vi "34401 - Config Measurement.vi"(0 "address":string, 1 "Manual Res. (1:5.5 Digits)":u16(ring)=1 items=["4.5 Digits", "5.5 Digits", "6.5 Digits"], 2 "Function (0:V DC)":u16(ring) items=["DC Voltage", "AC Voltage", "2--Wire Resistance", "4-Wire Resistance", "DC Current", "AC Current", "Frequency", "Period", "Continuity", "Diode Checking", "VDC: VDC Ratio"], 3 "AC Filter (1:Medium)":u16(ring)=1 items=["Slow", "Medium", "Fast"], 5 "Fixed DC Input Res. (T:On)":bool=TRUE, 7 "Manual Int. (0:Default)":u16(ring) items=["Default", "0.02 PLCs", "0.2 PLC", "1 PLCs", "10 PLCs", "100 PLCs"], 9 "Manual Apr. (0:Default)":u16(ring) items=["Default", "0.01 Sec", "0.1 Sec", "1 Sec"], 11 "error in (no error)":errorcluster, 12 "Ran/Res/Int/Apr (T:Auto)":bool=TRUE, 13 "Autozero (F:Off)":bool, 14 "Manual Range (0.00)":dbl min=0.0 format="%.2f") -> (15 "error out":errorcluster)   [LabVIEW 2014]
doc: "Configures the range, resolution, and other settings for the multimeter measurement."
panel:
  # "Auto"
  # "Manual"
  # "ON\nOFF"
  # "ON\nOFF"
  # "Note - Manually setting either the integration or aperture overrides the manual resolution settings."
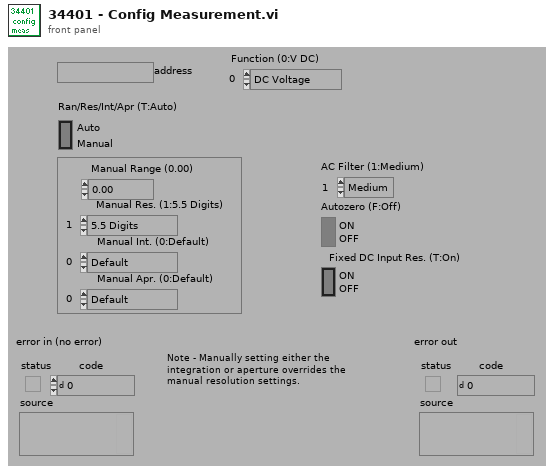
[diagram p1: front panel]
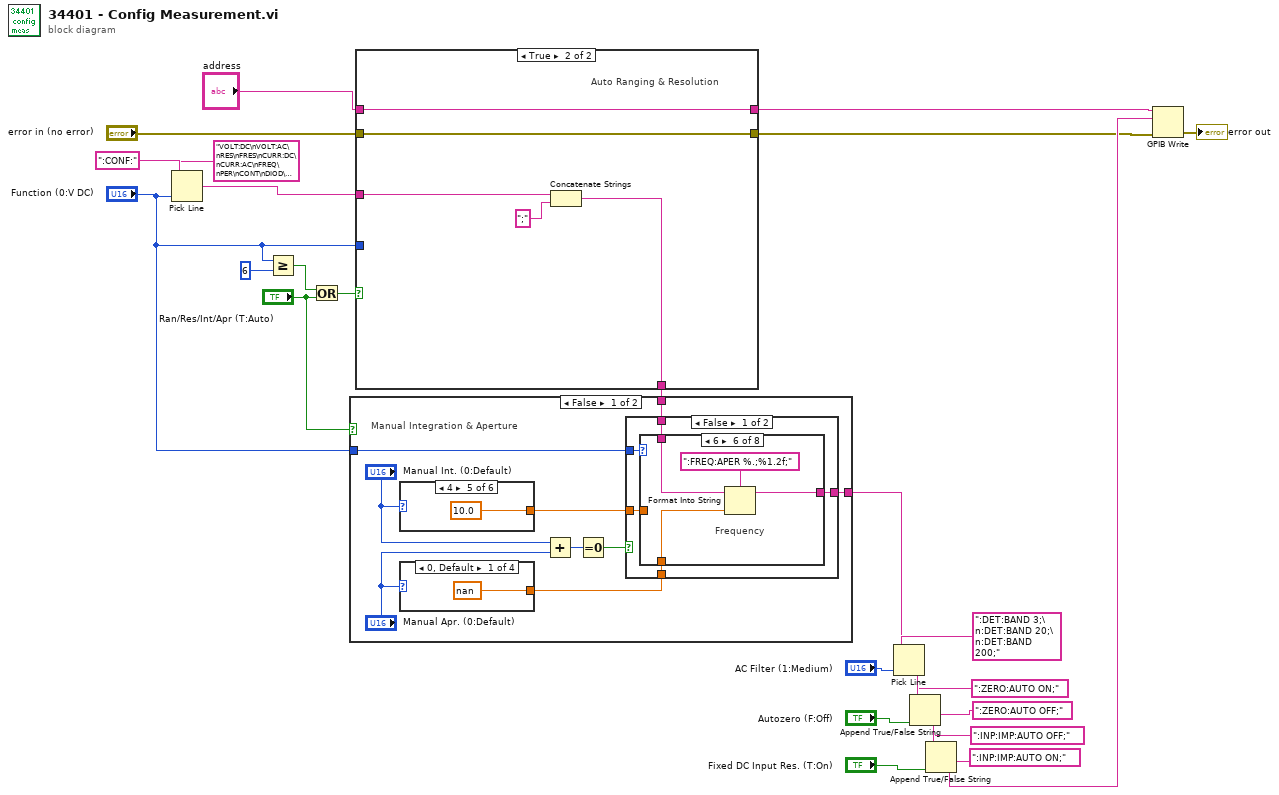
[diagram p0: block diagram]
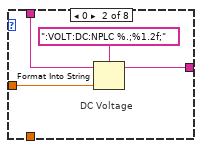
[diagram p3: hidden frame]
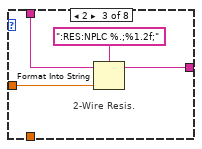
[diagram p4: hidden frame]
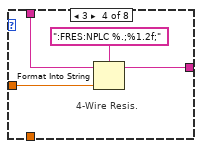
[diagram p5: hidden frame]
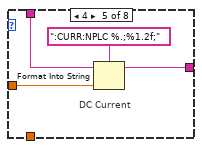
[diagram p6: hidden frame]
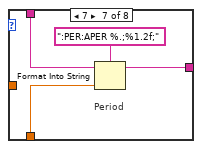
[diagram p7: hidden frame]
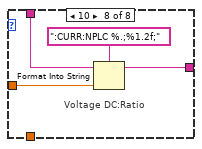
[diagram p8: hidden frame]
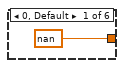
[diagram p10: hidden frame]
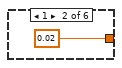
[diagram p11: hidden frame]
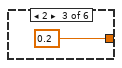
[diagram p12: hidden frame]
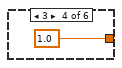
[diagram p13: hidden frame]
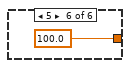
[diagram p14: hidden frame]
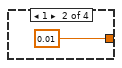
[diagram p15: hidden frame]
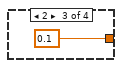
[diagram p16: hidden frame]
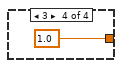
[diagram p17: hidden frame]
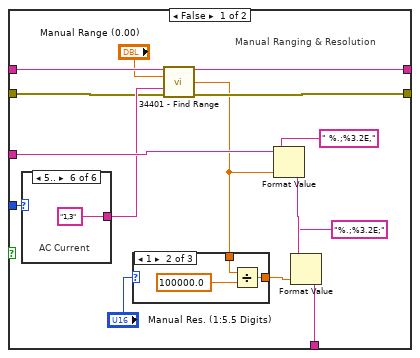
[diagram p19: hidden frame]
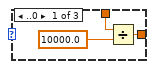
[diagram p20: hidden frame]
diagram:
  n1 = Pick Line(string ("")=":CONF:", multi-line string="VOLT:DC\nVOLT:AC\nRES\nFRES\nCURR:DC\nCURR:AC\nFREQ\nPER\nCONT\nDIOD\nVOLT:DC:RAT", line index="Function (0:V DC)") -> (output string=w21:string)
  n2 = Greater Or Equal?(x="Function (0:V DC)", y=u16 6) -> (x >= y?=w23:bool)
  n3 = Or(x=w23, y="Ran/Res/Int/Apr (T:Auto)") -> (x .or. y?=w22:bool)
  n4 = case shown="True" w22 {
    tunnel: w21 -> [w40 w61]
    tunnel: "Function (0:V DC)" -> [w41 _]
    tunnel: [w34 w59] -> w9
    tunnel: "error in (no error)" -> [w30 w58]
    tunnel: [w27 w57] -> w3
    tunnel: [w29 w58] -> w1
    tunnel: "address" -> [w33 w57]
    frame False {
      # "Manual Ranging & Resolution"
      n5 = case shown="5.." w41 {
        tunnel: [".1,1,10,100,1000" ".1,1,10,100,1000" "1E2,1E3,1E4,1E5,1E6,1E7,1E8" "1E2,1E3,1E4,1E5,1E6,1E7,1E8" ".01,.1,1,3" "1,3"] -> w31
        frame ..0 {
          # "DC Voltage"
        }
        frame 1 {
          # "AC Voltage"
        }
        frame 2 {
          # "2-Wire Resis."
        }
        frame 3 {
          # "4-Wire Resis."
        }
        frame 4 {
          # "DC Current"
        }
        frame 5.. {
          # "AC Current"
        }
      }
      n6 = call "34401 - Find Range.vi"("address"=w33, "Number to Range (0.00)"="Manual Range (0.00)", "Numeric Data (Empty)"=w31, "error in (no error)"=w30) -> ("dup address"=w27:string, "Ranged Number"=w28:dbl, "error out"=w29:errorcluster)  [unwired: 7 in, 2 out]
      n7 = case shown="1" "Manual Res. (1:5.5 Digits)" {
        tunnel: w28 -> [w43 w46 w49]
        tunnel: [w42 w45 w48] -> w38
        frame ..0 {
          n8 = Divide(x=w43, y=10000.0) -> (x/y=w42:dbl)
        }
        frame 1 {
          n9 = Divide(x=w46, y=100000.0) -> (x/y=w45:dbl)
        }
        frame 2.. {
          n10 = Divide(x=w49, y=1000000.0) -> (x/y=w48:dbl)
        }
      }
      n11 = Format Value(string ("")=w40, format string=" %.;%3.2E,", value (0)=w28) -> (output string=w39:string)
      n12 = Format Value(string ("")=w39, format string="%.;%3.2E;", value (0)=w38) -> (output string=w34:string)
    }
    frame True {
      # "Auto Ranging & Resolution"
      n13 = Concatenate Strings(w61, ";") -> (w59:string)
    }
  }
  n14 = case shown="False" "Ran/Res/Int/Apr (T:Auto)" {
    tunnel: w9 -> [w69 w116]
    tunnel: "Function (0:V DC)" -> [w67 _]
    tunnel: [w70 w116] -> w7
    frame False {
      # "Manual Integration & Aperture"
      n15 = case shown="4" "Manual Int. (0:Default)" {
        tunnel: [nan 0.02 0.2 1.0 10.0 100.0] -> w68
        frame 0, Default {
        }
        frame 1 {
        }
        frame 2 {
        }
        frame 3 {
        }
        frame 4 {
        }
        frame 5 {
        }
      }
      n16 = case shown="0, Default" "Manual Apr. (0:Default)" {
        tunnel: [nan 0.01 0.1 1.0] -> w66
        frame 0, Default {
        }
        frame 1 {
        }
        frame 2 {
        }
        frame 3 {
        }
      }
      n17 = Add(x="Manual Int. (0:Default)", y="Manual Apr. (0:Default)") -> (x+y=w63:u16)
      n18 = Equal To 0?(x=w63) -> (x = 0?=w62:bool)
      n19 = case shown="False" w62 {
        tunnel: [w75 w105] -> w70
        tunnel: w69 -> [w74 w105]
        tunnel: w68 -> [w73 _]
        tunnel: w67 -> [w72 _]
        tunnel: w66 -> [w71 _]
        frame False {
          n20 = case shown="6" w72 {
            tunnel: [w76 w79 w83 w87 w91 w93 w98 w103] -> w75
            tunnel: w74 -> [w76 w78 w82 w86 w90 w95 w99 w102]
            tunnel: w73 -> [_ w77 w81 w85 w89 _ _ w101]
            tunnel: w71 -> [_ _ _ _ _ w94 w97 _]
            frame Default {
              # "1 AC Voltage\n5 AC Current\n8 Continuity\n9 Diode Checking"
              # "Not Supported"
            }
            frame 0 {
              # "DC Voltage"
              n21 = Format Into String(format string=":VOLT:DC:NPLC %.;%1.2f;" ("Format String"), initial string=w78, w77) -> (resulting string=w79:string)  [unwired: 1 in, 1 out]
            }
            frame 2 {
              # "2-Wire Resis."
              n22 = Format Into String(format string=":RES:NPLC %.;%1.2f;" ("Format String"), initial string=w82, w81) -> (resulting string=w83:string)  [unwired: 1 in, 1 out]
            }
            frame 3 {
              # "4-Wire Resis."
              n23 = Format Into String(format string=":FRES:NPLC %.;%1.2f;" ("Format String"), initial string=w86, w85) -> (resulting string=w87:string)  [unwired: 1 in, 1 out]
            }
            frame 4 {
              # "DC Current"
              n24 = Format Into String(format string=":CURR:NPLC %.;%1.2f;" ("Format String"), initial string=w90, w89) -> (resulting string=w91:string)  [unwired: 1 in, 1 out]
            }
            frame 6 {
              # "Frequency"
              n25 = Format Into String(format string=":FREQ:APER %.;%1.2f;" ("Format String"), initial string=w95, w94) -> (resulting string=w93:string)  [unwired: 1 in, 1 out]
            }
            frame 7 {
              # "Period"
              n26 = Format Into String(format string=":PER:APER %.;%1.2f;" ("Format String"), initial string=w99, w97) -> (resulting string=w98:string)  [unwired: 1 in, 1 out]
            }
            frame 10 {
              # "Voltage DC:Ratio"
              n27 = Format Into String(format string=":CURR:NPLC %.;%1.2f;" ("Format String"), initial string=w102, w101) -> (resulting string=w103:string)  [unwired: 1 in, 1 out]
            }
          }
        }
        frame True {
          # "Not Selected"
        }
      }
    }
    frame True {
    }
  }
  n28 = Pick Line(string ("")=w7, multi-line string=":DET:BAND 3;\n:DET:BAND 20;\n:DET:BAND 200;", line index="AC Filter (1:Medium)") -> (output string=w20:string)
  n29 = Append True/False String(1:"Autozero (F:Off)", 2:":ZERO:AUTO OFF;", 3:":ZERO:AUTO ON;", 4:w20) -> (0:w14:string)
  n30 = Append True/False String(1:"Fixed DC Input Res. (T:On)", 2:":INP:IMP:AUTO ON;", 3:":INP:IMP:AUTO OFF;", 4:w14) -> (0:w2:string)
  n31 = GPIB Write(0:w3, 1:w2, 3:w1) -> (6:→"error out":errorcluster)  [unwired: 2 in, 1 out]
